vi "Send to DAQ.vi"(7 "Timeout (ms)":i32, 8 "error in (no error)":errorcluster, 9 "Send to DAQ?":bool, 10 "DAQ Message":T1, 11 "DAQ Communication in":refnum<class "DAQ Communication.lvclass">) -> (0 "error out":errorcluster, 3 "DAQ Communication out":refnum<class "DAQ Communication.lvclass">)   [LabVIEW 2026, in "TALOS.lvlib" / "Interfaces.lvlib" / "DAQ Communication.lvclass"]
uses:
  DAQ Communication.lvclass
  DAQ Message.ctl
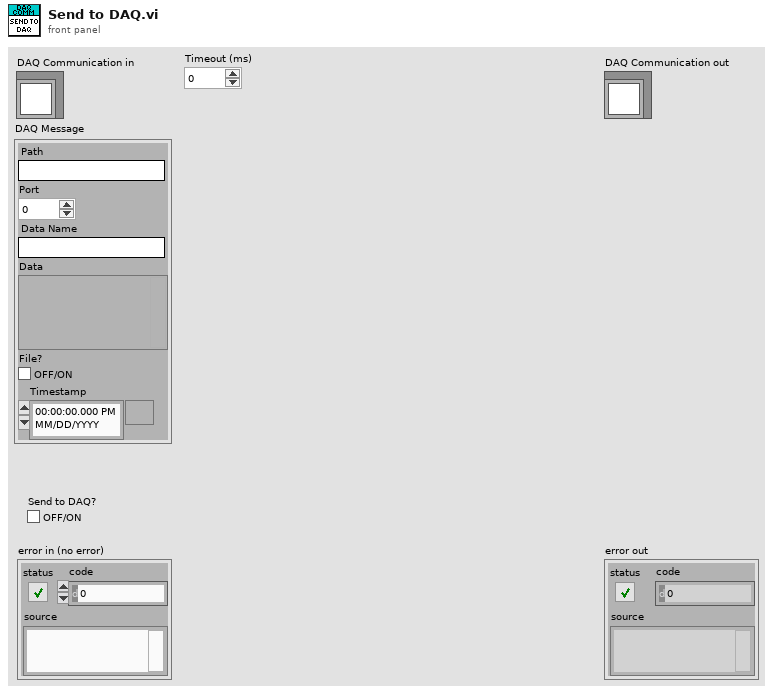
[diagram p1: front panel]
types:
  T1 = typedef "TALOS.lvlib/Interfaces.lvlib/DAQ Communication.lvclass/DAQ Message.ctl" = cluster{"Path":string, "Port":u16, "Data Name":string, "Data":variant, "File?":bool, "Timestamp":timestamp}
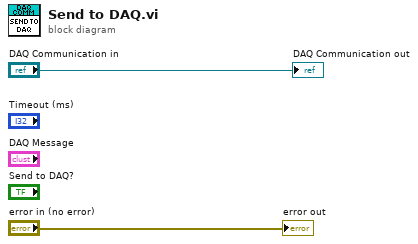
[diagram p0: block diagram]
diagram:
  "error out" <- "error in (no error)"
  "DAQ Communication out" <- "DAQ Communication in"
